vi "Generate Final Result.vi"(8 "error in (no error)":errorcluster, 11 "Results Manager in":refnum<class "Results Manager.lvclass">) -> (0 "error out":errorcluster, 2 "Array":T1[](array[typedef]), 3 "Results Manager out":refnum<class "Results Manager.lvclass">)   [LabVIEW 2021, in "Sequence Engine.lvlib" / "Results Manager.lvclass"]
uses:
  Results Manager.lvclass
  Test Result/Result Data.ctl
  Test Result/Test Status.ctl
  Results Manager.lvclass/Results Manager.ctl
  Test Result/Test Result.lvclass/Test Result.ctl
  Test Result/Test Result.lvclass
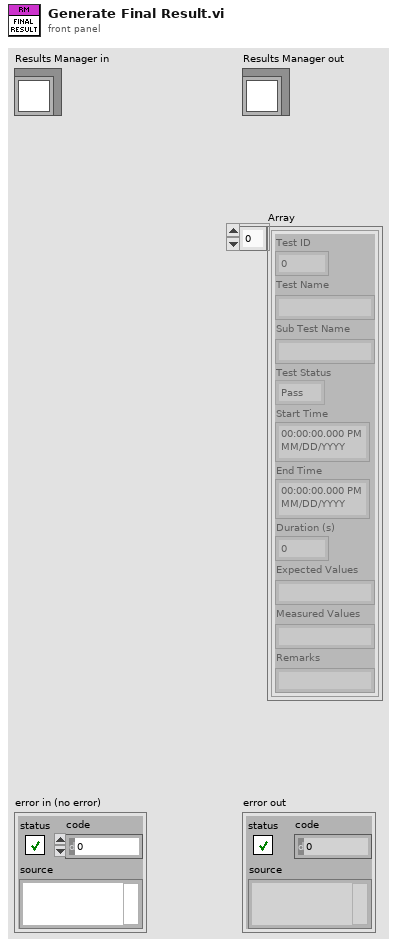
[diagram p1: front panel]
types:
  T1 = typedef "Sequence Engine.lvlib/Test Result.lvclass/Result Data.ctl" = cluster{"Test ID":u32, "Test Name":string, "Sub Test Name":string, "Test Status":T2, "Start Time":timestamp, "End Time":timestamp, "Duration (s)":dbl, "Expected Values":string, "Measured Values":string, "Remarks":string}
  T2 = typedef "Sequence Engine.lvlib/Test Result.lvclass/Test Status.ctl" = enum16{"Pass", "Fail", "Aborted", "Skipped"}
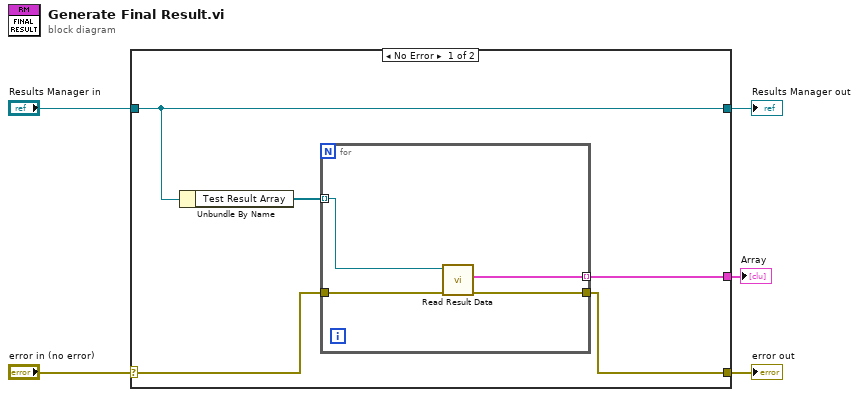
[diagram p0: block diagram]
diagram:
  n1 = case shown="No Error" "error in (no error)" {
    selector: "error in (no error)" -> [w7 w16]
    tunnel: [w6 w16] -> w4
    tunnel: [w10 w15] -> w2
    tunnel: "Results Manager in" -> [w10 w15]
    tunnel: [w8 _] -> w1
    frame No Error {
      n2 = Unbundle By Name(w10) -> ("Test Result Array"=w9:refnum<class "Test Result.lvclass">[])
      n3 = for {
        tunnel: w9 -> [w14] mode=indexing
        tunnel: [w13] -> w8 mode=indexing
        tunnel: w7 -> [w12]
        tunnel: [w11] -> w6
        n4 = call "Read Result Data.vi"("error in (no error)"=w12, "Test Result in"=w14) -> ("error out"=w11:errorcluster, "Result Data"=w13:T1)  [unwired: 7 in, 1 out]
      }
    }
    frame Error {
    }
  }
  "error out" <- w4
  "Results Manager out" <- w2
  "Array" <- w1
